vi "Compass Initialization_laptop.vi"(10 "Compass Initialization Parameters":T2={"VISA resource name"="COM1", "Baud Rate"=9600, "Compass Data Freq"=10}) -> (2 "Initialized Compass":T1)   [LabVIEW 2009]
uses:
  <vilib>/Instr/_visa.llb/VISA Set IO Buffer Mask.ctl
  <vilib>/Instr/_visa.llb/VISA Flush IO Buffer Mask.ctl
panel:
  in  "Cluster":T1
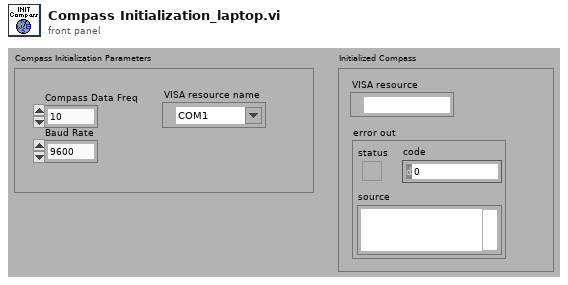
[diagram p1: front panel]
types:
  T1 = cluster{"VISA resource":refnum<visa-resource-name>, "error out":errorcluster}
  T2 = cluster{"VISA resource name":refnum<visa-resource-name>, "Baud Rate":i32, "Compass Data Freq":i32}
  T3 = typedef "VISA Set IO Buffer Mask.ctl" = u16
  T4 = typedef "VISA Flush IO Buffer Mask.ctl" = u16
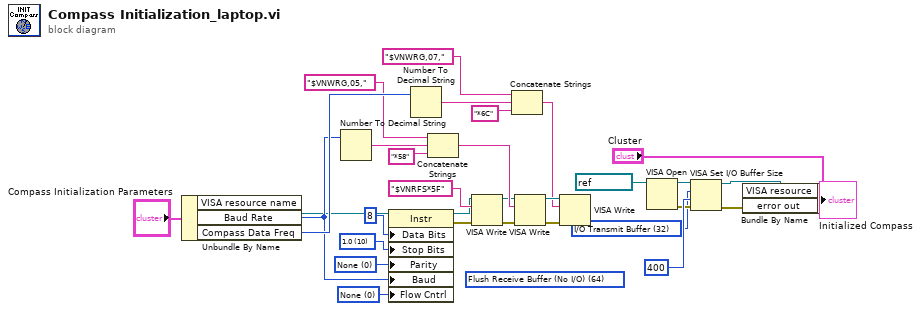
[diagram p0: block diagram]
diagram:
  w1 = T3 32 items=["I/O Receive Buffer"=16, "I/O Transmit Buffer"=32, "I/O Receive and Transmit Buffer"=48] ("Mask")
  (unwired) T4 64 items=["Flush Receive Buffer"=16, "Write Transmit Buffer to Device"=32, "Flush Receive Buffer (No I/O)"=64, "Flush Transmit Buffer"=128] ("Mask")
  w11 = u16 0 items=["None", "XON/XOFF", "RTS/CTS", "XON/XOFF & RTS/CTS", "DTR/DSR", "XON/XOFF & DTR/DSR"] ("Serial Settings:Flow Control")
  w13 = u16 10 items=["1.0"=10, "1.5"=15, "2.0"=20] ("Serial Settings:Stop Bits")
  w14 = u16 0 items=["None", "Odd", "Even", "Mark", "Space"] ("Serial Settings:Parity")
  n1 = Unbundle By Name("Compass Initialization Parameters") -> ("VISA resource name"=w10:refnum<visa-resource-name>, "Baud Rate"=w29:i32, "Compass Data Freq"=w31:i32)
  n2 = Number To Decimal String(number=w29) -> (decimal integer string=w26:string)  [unwired: 1 in]
  n3 = property class="Instr"(reference=w10, "Data Bits"=u16 8 ("Serial Settings:Data Bits"), "Stop Bits"=w13, "Parity"=w14, "Baud"=w29, "Flow Cntrl"=w11) -> (reference out=w9:refnum<visa-resource-name>, error out=w8:errorcluster)  [unwired: 1 in]
  n4 = Number To Decimal String(number=w31) -> (decimal integer string=w21:string)  [unwired: 1 in]
  n5 = Concatenate Strings("$VNWRG,05," ("string"), w26, "*58" ("string")) -> (w24:string)
  n6 = VISA Write(VISA resource name=w9, write buffer="$VNRFS*5F", error in (no error)=w8) -> (VISA resource name out=w18:refnum<visa-resource-name>, error out=w16:errorcluster)  [unwired: 1 out]
  n7 = Concatenate Strings("$VNWRG,07," ("string"), w21, "*6C" ("string")) -> (w15:string)
  n8 = VISA Write(VISA resource name=w18, write buffer=w24, error in (no error)=w16) -> (VISA resource name out=w20:refnum<visa-resource-name>, error out=w19:errorcluster)  [unwired: 1 out]
  n9 = VISA Write(VISA resource name=w20, write buffer=w15, error in (no error)=w19) -> ()  [unwired: 3 out]
  n10 = VISA Open(VISA resource name=refnum<visa-resource-name> "COM1" ("VISA resource")) -> (VISA resource name=w5:refnum<visa-resource-name>, error out=w3:errorcluster)  [unwired: 4 in]
  n11 = VISA Set I/O Buffer Size(VISA resource name=w5, mask (16)=w1, size (4096)=u32 400, error in (no error)=w3) -> (VISA resource name out=w4:refnum<visa-resource-name>, error out=w2:errorcluster)
  n12 = Bundle By Name(cluster="Cluster", "VISA resource"=w4, "error out"=w2) -> (→"Initialized Compass":T1)
